vi "Command Drive to Encoders.vi"(2 "Robot System Functions In":T1, 3 "Startup":bool, 4 "String Parameter":string, 5 "Cmd Parameter 3":dbl, 6 "Cmd Parameter 2":dbl, 7 "Cmd Parameter 1":dbl) -> (0 "Robot System Functions Out":T1, 1 "Completed":bool)   [LabVIEW 2016]
uses:
  Subsystems/All Robot Commands.ctl
  Subsystems/Drive and Climb SS/Drive + Climb Commands 2017.ctl
  Subsystems/Gear Delivery SS/Gear Delivery Commands.ctl
  Subsystems/Conveyor and Shooter SS/Conveyor and Shooter Commands.ctl
  Subsystems/Ball Intake SS/Ball Intake Commands.ctl
  Command Execution State.ctl
  <vilib>/Rock Robotics/WPI/ThirdParty/CanMotor/TalonSRX/WPI_CANTalonSRX_APIControlMode.ctl
  Global Variables/Refnum Names.vi
  Global Variables/Auto Drive Calibrations.vi
  Global Variables/Sensor Data.vi
panel:
  out "Right F":dbl
  out "Right D":dbl
  out "Right I":dbl
  out "Right P":dbl
  out "Left F":dbl
  out "Left D":dbl
  out "Left I":dbl
  out "Left P":dbl
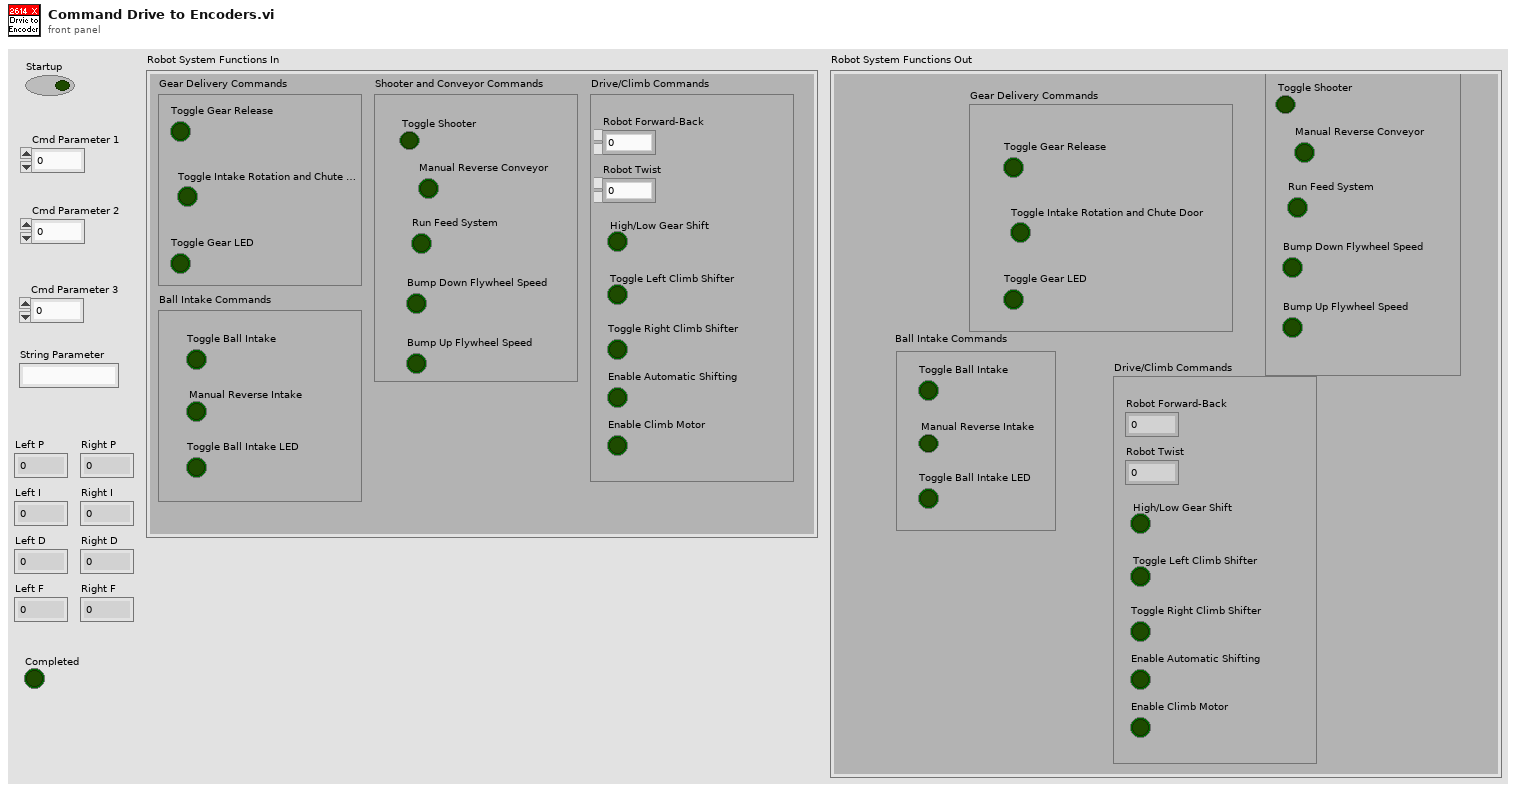
[diagram p1: front panel]
types:
  T1 = typedef "All Robot Commands.ctl" = cluster{"Drive/Climb Commands":T2, "Gear Delivery Commands":T3, "Shooter and Conveyor Commands":T4, "Ball Intake Commands":T5}
  T2 = typedef "Drive + Climb Commands 2017.ctl" = cluster{"Robot Forward-Back":dbl, "Robot Twist":dbl, "High/Low Gear Shift":bool, "Toggle Left Climb Shifter":bool, "Toggle Right Climb Shifter":bool, "Enable Automatic Shifting":bool, "Enable Climb Motor ":bool}
  T3 = typedef "Gear Delivery Commands.ctl" = cluster{"Toggle Gear Release":bool, "Toggle Intake Rotation and Chute Door":bool, "Toggle Gear LED":bool}
  T4 = typedef "Conveyor and Shooter Commands.ctl" = cluster{"Toggle Shooter":bool, "Manual Reverse Conveyor":bool, "Run Feed System":bool, "Bump Down Flywheel Speed":bool, "Bump Up Flywheel Speed":bool}
  T5 = typedef "Ball Intake Commands.ctl" = cluster{"Toggle Ball Intake":bool, "Manual Reverse Intake":bool, "Toggle Ball Intake LED":bool}
  T6 = typedef "Command Execution State.ctl" = enum16{"Initialize", "Execute", "Finish"}
  T7 = typedef "WPI_CANTalonSRX_APIControlMode.ctl" = enum8{"Percent VBus", "Speed", "Position", "Slave", "Unchanged / Invalid", "Voltage Compensation", "Current", "Motion Profile", "Motion Magic"}
  T8 = typedef "WPI_MotorControlDeviceRef.ctl" = cluster{"DeviceStatus":errorcluster, "Type":T9, "PWM":cluster{"PWM Channel":T10, "DeadBand":T11}, "CAN":cluster{"Device Number":u8, "SetOutput VI Ref":variant, "GetOutput VI Ref":variant, "Enable VI Ref":variant, "Disable VI Ref":variant, "Data":variant}, "Invert":bool}
  T9 = typedef "WPI_MotorControlType.ctl" = enum16{"PWM", "CAN"}
  T10 = typedef "FPGA_DIOPWMChannel.ctl" = enum8{"PWM 0", "PWM 1", "PWM 2", "PWM 3", "PWM 4", "PWM 5", "PWM 6", "PWM 7", "PWM 8", "PWM 9", "PWM MXP 0", "PWM MXP 1", "PWM MXP 2", "PWM MXP 3", "PWM MXP 4", "PWM MXP 5", "PWM MXP 6", "PWM MXP 7", "PWM MXP 8", "PWM MXP 9", "Invalid"}
  T11 = typedef "WPI_PWMDeadband.ctl" = cluster{"Name":string, "maxPositivePwm":i32, "minPositivePwm":i32, "centerPwm":i32, "maxNegativePwm":i32, "minNegativePwm":i32, "angularRange":u16}
  T12 = cluster{"Goal":dbl, "Process Variable":dbl, "Max Ouput":dbl, dbl, dbl, dbl, dbl}
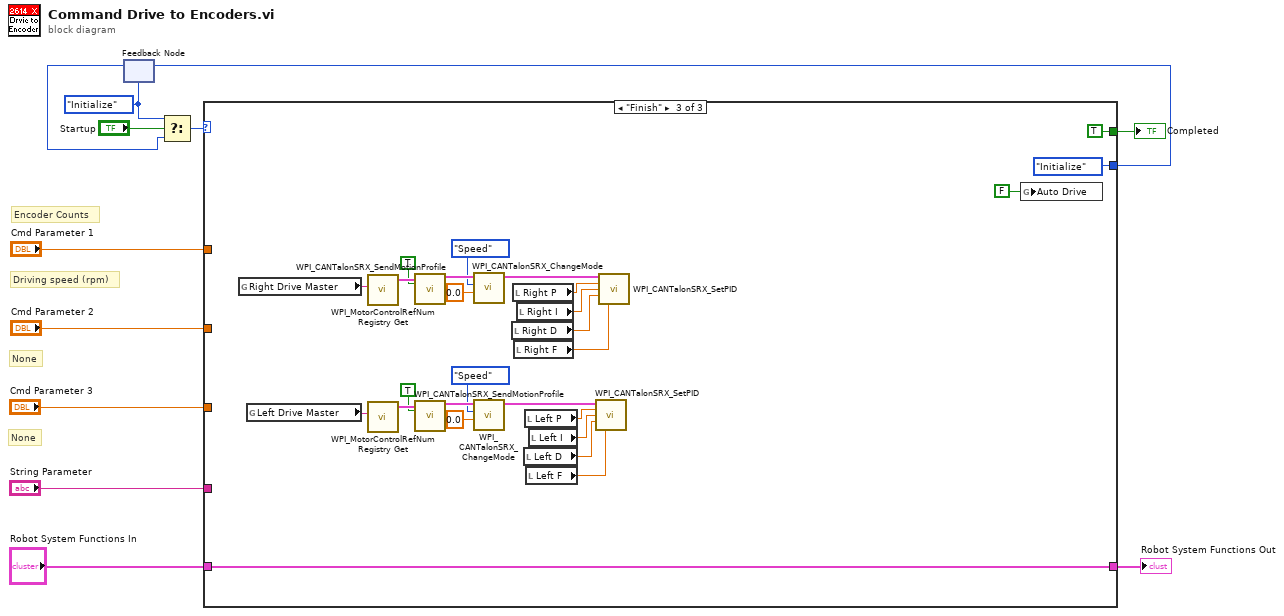
[diagram p0: block diagram]
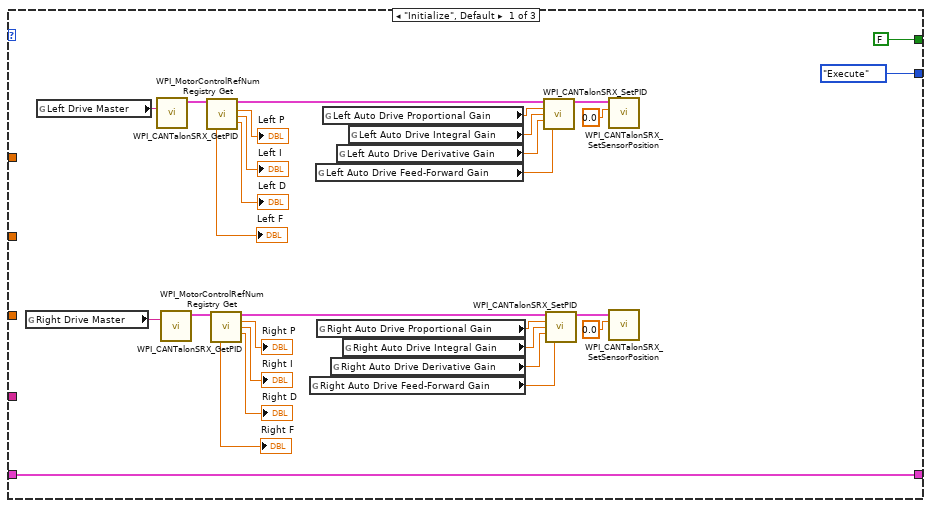
[diagram p2: hidden frame]
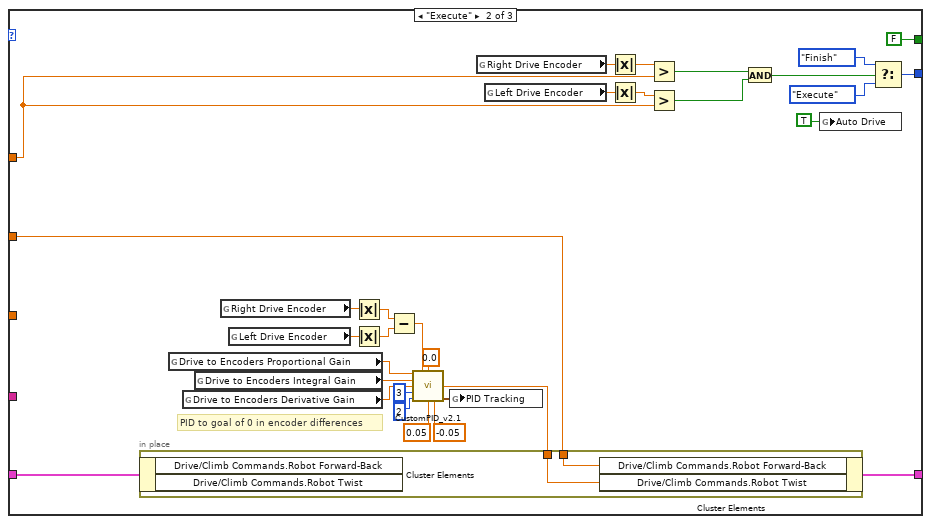
[diagram p3: hidden frame]
diagram:
  w7 = Command_Execution_State."Initialize" ("Play State")
  # "None"
  # "None"
  # "Driving speed (rpm)"
  # "Encoder Counts"
  n1 = feedback #1(w7) -> (w8:T6)
  n2 = Select(t=w7, s="Startup", f=w8) -> (s? t:f=w12:T6)
  n3 = case shown="\"Finish\"" w12 {
    tunnel: [FALSE FALSE TRUE] -> w10
    tunnel: [Command_Execution_State."Execute" ("Play State") w70 Command_Execution_State."Initialize" ("f")] -> w9
    tunnel: "Cmd Parameter 1" -> [_ w54 _]
    tunnel: "Cmd Parameter 2" -> [_ w42 _]
    tunnel: [w23 w67 w98] -> w4
    tunnel: "Robot System Functions In" -> [w23 w68 w98]
    tunnel: "Cmd Parameter 3" -> [_ _ _]
    tunnel: "String Parameter" -> [_ _ _]
    frame "Initialize", Default {
      n4 = global read "Refnum Names.vi" "Right Drive Master"() -> (w33:string)
      n5 = global read "Refnum Names.vi" "Left Drive Master"() -> (w39:string)
      n6 = call <vilib>:"WPI_MotorControlRefNum Registry Get.vi"("refnum name"=w39) -> ("MotorControlDevRef"=w38:T8)  [unwired: 9 in, 1 out]
      n7 = call <vilib>:"WPI_MotorControlRefNum Registry Get.vi"("refnum name"=w33) -> ("MotorControlDevRef"=w32:T8)  [unwired: 9 in, 1 out]
      n8 = call <vilib>:"WPI_CANTalonSRX_GetPID.vi"("CAN Talon SRX Ref"=w38) -> ("CAN Talon SRX Ref"=w13:T8, "P"=→"Left P":dbl, "I"=→"Left I":dbl, "D"=→"Left D":dbl, "F"=→"Left F":dbl)  [unwired: 7 in, 3 out]
      n9 = call <vilib>:"WPI_CANTalonSRX_GetPID.vi"("CAN Talon SRX Ref"=w32) -> ("CAN Talon SRX Ref"=w25:T8, "P"=→"Right P":dbl, "I"=→"Right I":dbl, "D"=→"Right D":dbl, "F"=→"Right F":dbl)  [unwired: 7 in, 3 out]
      n10 = global read "Auto Drive Calibrations.vi" "Right Auto Drive Feed-Forward Gain"() -> (w20:dbl)
      n11 = global read "Auto Drive Calibrations.vi" "Left Auto Drive Feed-Forward Gain"() -> (w15:dbl)
      n12 = global read "Auto Drive Calibrations.vi" "Right Auto Drive Proportional Gain"() -> (w19:dbl)
      n13 = global read "Auto Drive Calibrations.vi" "Left Auto Drive Proportional Gain"() -> (w18:dbl)
      n14 = global read "Auto Drive Calibrations.vi" "Right Auto Drive Derivative Gain"() -> (w21:dbl)
      n15 = global read "Auto Drive Calibrations.vi" "Left Auto Drive Derivative Gain"() -> (w16:dbl)
      n16 = global read "Auto Drive Calibrations.vi" "Right Auto Drive Integral Gain"() -> (w22:dbl)
      n17 = global read "Auto Drive Calibrations.vi" "Left Auto Drive Integral Gain"() -> (w17:dbl)
      n18 = call <vilib>:"WPI_CANTalonSRX_SetPID.vi"("CAN Talon SRX Ref"=w13, "P"=w18, "I"=w17, "D"=w16, "F"=w15) -> ("CAN Talon SRX Ref"=w14:T8)  [unwired: 9 in, 1 out]
      n19 = call <vilib>:"WPI_CANTalonSRX_SetPID.vi"("CAN Talon SRX Ref"=w25, "P"=w19, "I"=w22, "D"=w21, "F"=w20) -> ("CAN Talon SRX Ref"=w24:T8)  [unwired: 9 in, 1 out]
      n20 = call <vilib>:"WPI_CANTalonSRX_SetSensorPosition.vi"("New Sensor Position"=0.0, "CAN Talon SRX Ref"=w14) -> ()  [unwired: 8 in, 2 out]
      n21 = call <vilib>:"WPI_CANTalonSRX_SetSensorPosition.vi"("New Sensor Position"=0.0, "CAN Talon SRX Ref"=w24) -> ()  [unwired: 8 in, 2 out]
    }
    frame "Execute" {
      # "PID to goal of 0 in encoder differences"
      n22 = global read "Auto Drive Calibrations.vi" "Drive to Encoders Proportional Gain"() -> (w45:dbl)
      n23 = global read "Auto Drive Calibrations.vi" "Drive to Encoders Derivative Gain"() -> (w43:dbl)
      n24 = global read "Auto Drive Calibrations.vi" "Drive to Encoders Integral Gain"() -> (w44:dbl)
      n25 = global read "Sensor Data.vi" "Right Drive Encoder"() -> (w50:dbl)
      n26 = global read "Sensor Data.vi" "Left Drive Encoder"() -> (w49:dbl)
      n27 = Absolute Value(x=w50) -> (abs(x)=w47:dbl)
      n28 = Absolute Value(x=w49) -> (abs(x)=w48:dbl)
      n29 = Subtract(x=w47, y=w48) -> (x-y=w46:dbl)
      n30 = call "CustomPID_v2.1.vi"("Kp"=w45, "Process Variable"=w46, "Goal"=0.0, "Ki"=w44, "Kd"=w43, "N-Diff"=3, "N-Int"=2, "Max Ouput"=0.05, "Min Output"=-0.05) -> ("Command"=w57:dbl, "PID Tracking"=w51:T12)  [unwired: 4 in, 1 out]
      n31 = in-place {
        in-place-border: w57 -> [w74]
        in-place-border: w42 -> [w73]
        n32 = in-place-cluster #2(w68) -> ()  [unwired: 2 out]
        n33 = in-place-cluster #2("Drive/Climb Commands.Robot Forward-Back"=w73, "Drive/Climb Commands.Robot Twist"=w74) -> (w67:T1)
      }
      n34 = global write "Auto Drive Calibrations.vi" "PID Tracking"(w51) -> ()
      n35 = global read "Sensor Data.vi" "Right Drive Encoder"() -> (w59:dbl)
      n36 = global read "Sensor Data.vi" "Left Drive Encoder"() -> (w56:dbl)
      n37 = Absolute Value(x=w59) -> (abs(x)=w58:dbl)
      n38 = Absolute Value(x=w56) -> (abs(x)=w55:dbl)
      n39 = Greater?(x=w58, y=w54) -> (0:w60:bool)
      n40 = Greater?(x=w55, y=w54) -> (0:w61:bool)
      n41 = And(x=w60, y=w61) -> (x .and. y?=w53:bool)
      n42 = global write "Auto Drive Calibrations.vi" "Auto Drive"(TRUE ("PID Heading")) -> ()
      n43 = Select(t=Command_Execution_State."Finish" ("Play State"), s=w53, f=Command_Execution_State."Execute") -> (s? t:f=w70:T6)
    }
    frame "Finish" {
      n44 = global read "Refnum Names.vi" "Right Drive Master"() -> (w77:string)
      n45 = global read "Refnum Names.vi" "Left Drive Master"() -> (w88:string)
      n46 = call <vilib>:"WPI_MotorControlRefNum Registry Get.vi"("refnum name"=w77) -> ("MotorControlDevRef"=w82:T8)  [unwired: 9 in, 1 out]
      n47 = call <vilib>:"WPI_MotorControlRefNum Registry Get.vi"("refnum name"=w88) -> ("MotorControlDevRef"=w93:T8)  [unwired: 9 in, 1 out]
      n48 = call <vilib>:"WPI_CANTalonSRX_SendMotionProfile.vi"("CAN Talon SRX Ref"=w82, "Clear"=TRUE) -> ("CAN Talon SRX Ref Out"=w79:T8)  [unwired: 10 in, 3 out]
      n49 = call <vilib>:"WPI_CANTalonSRX_SendMotionProfile.vi"("CAN Talon SRX Ref"=w93, "Clear"=TRUE) -> ("CAN Talon SRX Ref Out"=w90:T8)  [unwired: 10 in, 3 out]
      n50 = call <vilib>:"WPI_CANTalonSRX_ChangeMode.vi"("Output"=0.0, "Control Mode"=WPI_CANTalonSRX_APIControlMode."Speed", "CAN Talon SRX Ref"=w79) -> ("CAN Talon SRX Ref"=w76:T8)  [unwired: 7 in, 1 out]
      n51 = call <vilib>:"WPI_CANTalonSRX_ChangeMode.vi"("Output"=0.0, "Control Mode"=WPI_CANTalonSRX_APIControlMode."Speed", "CAN Talon SRX Ref"=w90) -> ("CAN Talon SRX Ref"=w87:T8)  [unwired: 7 in, 1 out]
      n52 = local read "Right D"() -> (w95:dbl)
      n53 = local read "Right P"() -> (w97:dbl)
      n54 = local read "Right F"() -> (w94:dbl)
      n55 = local read "Right I"() -> (w96:dbl)
      n56 = local read "Left D"() -> (w84:dbl)
      n57 = local read "Left P"() -> (w86:dbl)
      n58 = local read "Left F"() -> (w83:dbl)
      n59 = local read "Left I"() -> (w85:dbl)
      n60 = call <vilib>:"WPI_CANTalonSRX_SetPID.vi"("CAN Talon SRX Ref"=w87, "P"=w86, "I"=w85, "D"=w84, "F"=w83) -> ()  [unwired: 9 in, 2 out]
      n61 = call <vilib>:"WPI_CANTalonSRX_SetPID.vi"("CAN Talon SRX Ref"=w76, "P"=w97, "I"=w96, "D"=w95, "F"=w94) -> ()  [unwired: 9 in, 2 out]
      n62 = global write "Auto Drive Calibrations.vi" "Auto Drive"(FALSE ("PID Heading")) -> ()
    }
  }
  "Completed" <- w10
  "Robot System Functions Out" <- w4
  n63 = feedback-in #1(w9) -> ()
